vi "SendFirebase.vi"() -> ()   [LabVIEW 2022 SP3]
uses:
  <vilib>/httpClient/PUTBuffer.vi
  <vilib>/httpClient/LabVIEWHTTPClient.lvlib
panel:
  out "String 2":string
  in  "Numbers":cluster{"Test":dbl}
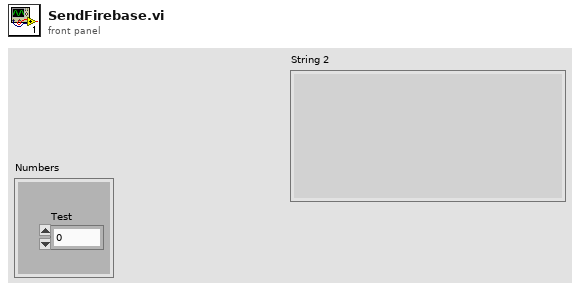
[diagram p1: front panel]
types:
  T1 = typedef "LabVIEWHTTPClient.lvlib/ClientHandle.ctl" = refnum<k1>
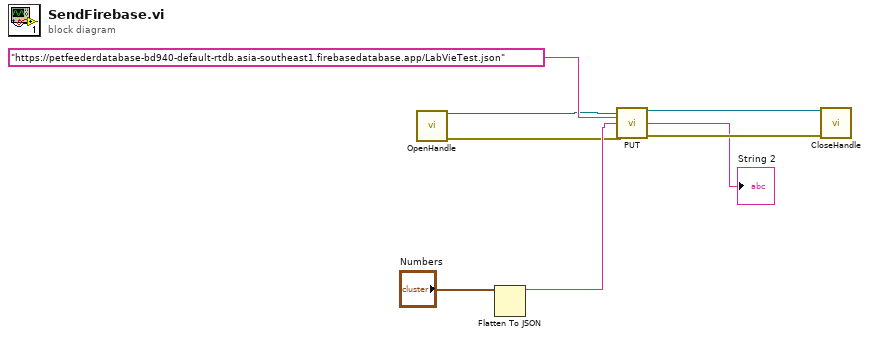
[diagram p0: block diagram]
diagram:
  n1 = call <vilib>:"OpenHandle.vi"() -> ("client handle out"=w5:T1, "error out"=w3:errorcluster)  [unwired: 14 in]
  n2 = Flatten To JSON(anything="Numbers") -> (JSON string=w7:string)  [unwired: 2 in, 1 out]
  n3 = call-poly <vilib>:"PUT.vi"("client handle"=w5, "url"="https://petfeederdatabase-bd940-default-rtdb.asia-southeast1.firebasedatabase.app/LabVieTest.json", "buffer"=w7, "error in (no error)"=w3) -> ("client handle out"=w4:T1, "body"=→"String 2":string, "error out"=w2:errorcluster)  [unwired: 8 in, 1 out]
  n4 = call <vilib>:"CloseHandle.vi"("client handle"=w4, "error in (no error)"=w2) -> ()  [unwired: 13 in, 1 out]
